vi "IK3.vi"(8 "L1":dbl=80.0, 10 "L2":dbl=80.0, 11 "coordinates":cluster{"x":dbl, "y":dbl}) -> (0 "theta31":dbl, 1 "theta21":dbl, 2 "theta11":dbl)   [LabVIEW 2024]
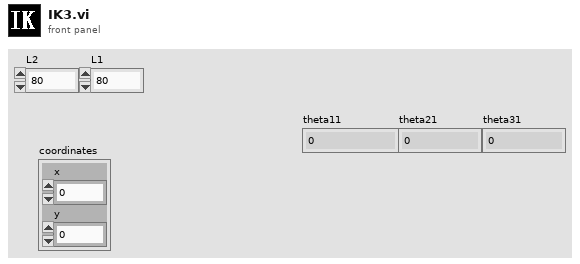
[diagram p1: front panel]
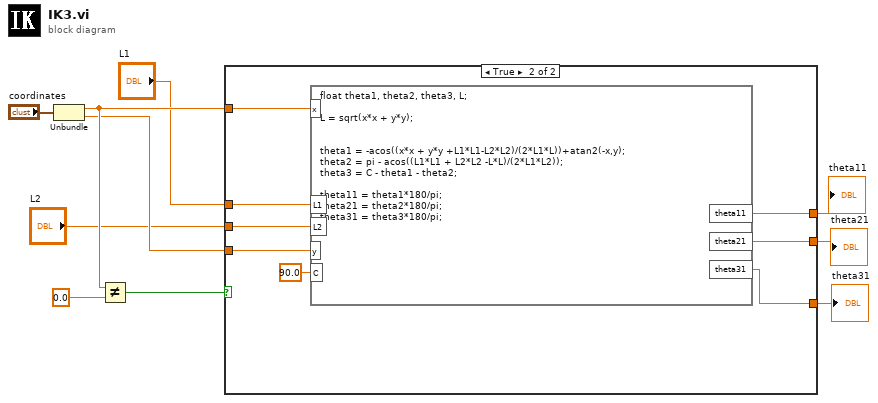
[diagram p0: block diagram]
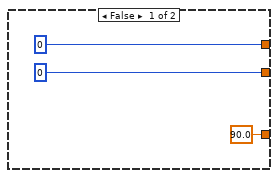
[diagram p2: hidden frame]
diagram:
  n1 = Unbundle("coordinates") -> ("x"=w10:dbl, "y"=w7:dbl)
  n2 = Not Equal?(x=w10, y=0.0) -> (x != y?=w8:bool)
  n3 = case shown="True" w8 {
    tunnel: "L1" -> [_ w21]
    tunnel: "L2" -> [_ w20]
    tunnel: [0 w19] -> w5
    tunnel: [0 w18] -> w4
    tunnel: w10 -> [_ w17]
    tunnel: w7 -> [_ w16]
    tunnel: [90.0 ("theta31") w15] -> w1
    frame False {
    }
    frame True {
      n4 = formula code="float theta1, theta2, theta3, L;\n\nL = sqrt(x*x + y*y);\n\n\ntheta1 = -acos((x*x + y*y +L1*L1-L2*L2)/(2*L1*L))+atan2(-x,y);\ntheta2 = pi - acos((L1*L1 + L2*L2 -L*L)/(2*L1*L2));\ntheta3 = C - theta1 - theta2;\n\ntheta11 = theta1*180/pi;\ntheta21 = theta2*180/pi;\ntheta31 = theta3*180/pi;"("L1"=w21, "L2"=w20, "x"=w17, "y"=w16, "C"=90.0 ("input variable")) -> ("theta11"=w19:dbl, "theta21"=w18:dbl, "theta31"=w15:dbl)
    }
  }
  "theta11" <- w5
  "theta21" <- w4
  "theta31" <- w1
